vi "BRig_dataBlock_c_nWrong_total.vi"() -> (2 "output_c_nWrong_total":i32)   [LabVIEW 2014]
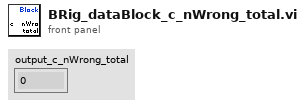
[diagram p1: front panel]
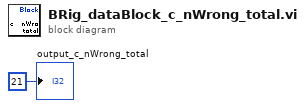
[diagram p0: block diagram]
diagram:
  "output_c_nWrong_total" <- 21 ("output_iBlock")
